vi "Scan units and defaults.vi"(0 "Name [Units] (default value)":string, 1 "Array Position (none)":i32[](array[numeric]), 2 "Default from text? (F)":bool, 5 "Default":variant, 7 "Classname":string, 9 "Type":T2, 11 "error in":errorcluster, 12 "Faultable (F)":bool, 14 "Scalable (F)":bool) -> (6 "Name out":string, 10 "Channel":T1, 15 "error out":errorcluster)   [LabVIEW 2016, in "DCM System Explorer.lvlib"]
uses:
  DCM System Explorer.lvlib
  <vilib>/NI Veristand/Custom Device API/Custom Device Channel Type.ctl
  <vilib>/NI Veristand/Custom Device API/Custom Device Channel.ctl
  <vilib>/NI VeriStand/Custom Device API/Custom Device API.lvlib
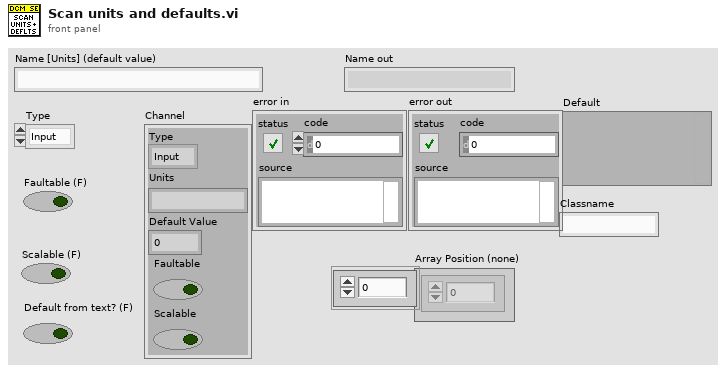
[diagram p1: front panel]
types:
  T1 = typedef "Custom Device API.lvlib/Custom Device Channel.ctl" = cluster{"Type":T2, "Units":string, "Default Value":dbl, "Faultable":bool, "Scalable":bool}
  T2 = typedef "Custom Device API.lvlib/Custom Device Channel Type.ctl" = enum16{"Input", "Output"}
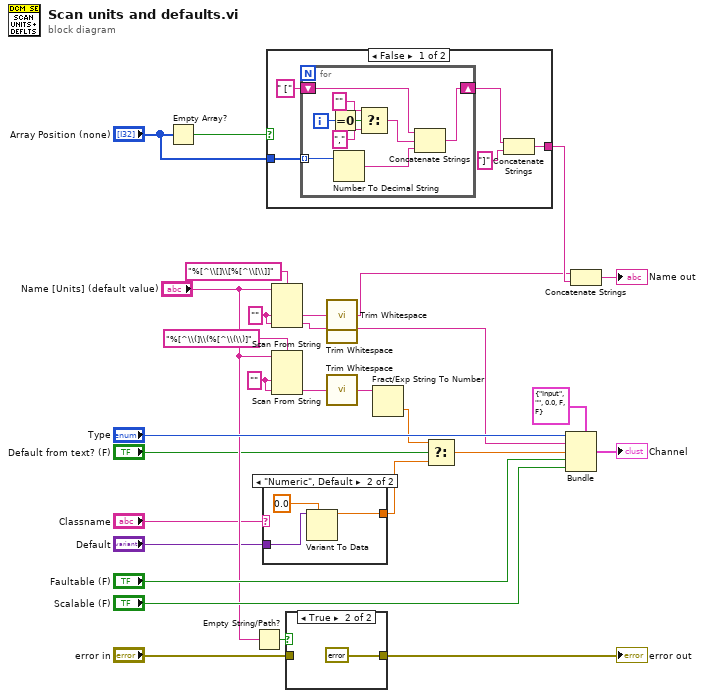
[diagram p0: block diagram]
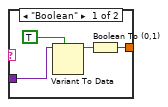
[diagram p2: hidden frame]
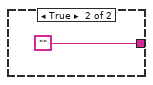
[diagram p4: hidden frame]
diagram:
  w12 = "" ("default value 2")
  w20 = "" ("default value 2")
  n1 = Empty Array?(array="Array Position (none)") -> (empty?=w24:bool)
  n2 = Empty String/Path?(string/path="Name [Units] (default value)") -> (empty?=w10:bool)
  n3 = case shown="\"Numeric\", Default" "Classname" {
    tunnel: "Default" -> [w33 w36]
    tunnel: [w30 w34] -> w2
    frame "Boolean" {
      n4 = Variant To Data(type=TRUE, Variant=w33) -> (data=w31:bool)  [unwired: 1 in, 1 out]
      n5 = Boolean To (0,1)(Boolean=w31) -> (0, 1=w30:i16)
    }
    frame "Numeric", Default {
      n6 = Variant To Data(type=0.0, Variant=w36) -> (data=w34:dbl)  [unwired: 1 in, 1 out]
    }
  }
  n7 = case shown="False" w24 {
    tunnel: "Array Position (none)" -> [w41 _]
    tunnel: [w38 ""] -> w21
    frame False {
      n8 = for {
        tunnel: w41 -> [w50] mode=indexing
        shift-right: [w49] -> w39
        shift-left: " [" -> [w47]
        i -> [w42]
        n9 = Equal To 0?(x=w42) -> (x = 0?=w44:bool)
        n10 = Number To Decimal String(number=w50) -> (decimal integer string=w48:string)  [unwired: 1 in]
        n11 = Select(t="" ("string"), s=w44, f="," ("string")) -> (s? t:f=w43:string)
        n12 = Concatenate Strings(w47, w43, w48) -> (w49:string)
      }
      n13 = Concatenate Strings(w39, "]" ("string")) -> (w38:string)
    }
    frame True {
    }
  }
  n14 = Scan From String(format string="%[^\\[]\\[%[^\\[\\]]" ("regular expression"), input string="Name [Units] (default value)", default 1=w20, default 2=w20) -> (output 1=w18:string, output 2=w16:string)  [unwired: 2 in, 3 out]
  n15 = Scan From String(format string="%[^\\(]\\(%[^\\(\\)]" ("regular expression"), input string="Name [Units] (default value)", default 1=w12, default 2=w12) -> (output 2=w11:string)  [unwired: 3 in, 3 out]
  n16 = case shown="True" w10 {
    tunnel: "error in" -> [w52 _]
    tunnel: [w52 errorcluster {"status"=TRUE, "code"=1, "source"="Scan From String (arg 1) in DCM-2116 Custom Device System Explorer.lvlib:Scan units and defaults.vi"} ("error out")] -> w7
    frame False {
    }
    frame True {
    }
  }
  "error out" <- w7
  n17 = call <vilib>:"Trim Whitespace.vi"("string"=w18) -> ("trimmed string"=w17:string)  [unwired: 1 in]
  n18 = call <vilib>:"Trim Whitespace.vi"("string"=w16) -> ("trimmed string"=w15:string)  [unwired: 1 in]
  n19 = call <vilib>:"Trim Whitespace.vi"("string"=w11) -> ("trimmed string"=w14:string)  [unwired: 1 in]
  n20 = Fract/Exp String To Number(string=w14) -> (number=w5:dbl)  [unwired: 3 in, 1 out]
  n21 = Select(t=w5, s="Default from text? (F)", f=w2) -> (s? t:f=w1:dbl)
  n22 = Bundle(cluster=T1 {"Type"=enum."Input", "Units"="", "Default Value"=0.0, "Faultable"=FALSE, "Scalable"=FALSE} ("Channel"), "Type"="Type", "Units"=w15, "Default Value"=w1, "Faultable"="Faultable (F)", "Scalable"="Scalable (F)") -> (→"Channel":T1)
  n23 = Concatenate Strings(w17, w21) -> (→"Name out":string)
